vi "Destroy ProjectBuilder.vi"(0 "reference in":refnum<class "ProjectBuilder.lvclass">, 5 "error in (no error)":errorcluster) -> (14 "reference out":refnum<class "ProjectBuilder.lvclass">, 19 "error out":errorcluster)   [LabVIEW 2015, in "ProjectBuilder.lvclass"]
uses:
  ProjectBuilder.lvclass
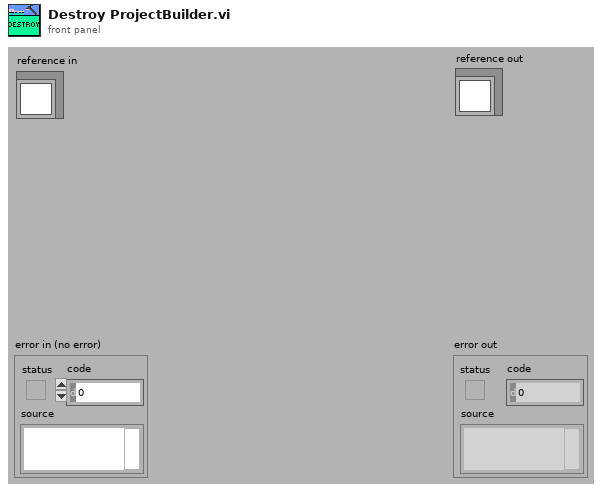
[diagram p1: front panel]
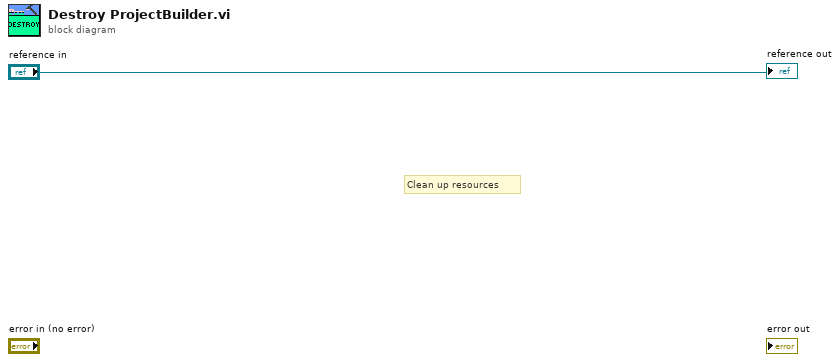
[diagram p0: block diagram]
diagram:
  # "Clean up resources"
  "reference out" <- "reference in"
